vi "Main.vi"(11 "Module Admin":refnum<class "Delacor_lib_QMH_Module Admin.lvclass">) -> ()   [LabVIEW 2024, in "Settings Editor.lvlib"]
doc: "This template is based off of the Queued Message Handler design pattern and the Queued Message Handler project template that ships with LabVIEW.\n\nThe main difference is that the queue is private to this module and communication between modules is performed via Broadcast and Request events.\n\nRequest events are wrapped in public API methods and are handled in the Event Handling Loop (EHL) of this VI. Any module can register for Broadcast events sent by this module. The EHL generates messages based on user interface actions.\n\nThe Message Handling Loop (MHL) processes messages generated by the EHL, or by other messages. The messages are string values, so new messages can be added easily to the Message Cases case structure in the MHL. Each message cluster can also provide an optional value for Message Data, which is a variant that can be converted to whatever message-specific data is required.\n_____\nBased on DQMH Project Template 4.0.0.47.\n_____\nBased on DQMH Dev Tools: Project Template 7.1.0.1503."
uses:
  Settings Editor.lvlib
  <vilib>/Delacor/Delacor QMH/Libraries/Module Admin_class/Delacor_lib_QMH_Module Admin.lvclass
  CML Shared/Signal Type--enum.ctl
  CML Shared/Calibration Values--cluster.ctl
  Module Data--cluster.ctl
  Settings--cluster.ctl
  Stop Argument--cluster.ctl
  <vilib>/Delacor/Delacor QMH/Libraries/Message Queue_class/Delacor_lib_QMH_Message Queue.lvclass/Delacor_lib_QMH_Message Queue.ctl
  Update Application Settings Argument--cluster.ctl
  Update Application Settings (Reply Payload)--cluster.ctl
  <vilib>/Delacor/Delacor QMH/Libraries/Module Admin_class/Delacor_lib_QMH_Module Admin.lvclass/Delacor_lib_QMH_Module Admin.ctl
  <vilib>/Utility/miscctls.llb/LVPointTypeDef.ctl
  <vilib>/Delacor/Delacor QMH/Libraries/Message Queue_class/Delacor_lib_QMH_Enqueue Message (Single).vi
  <vilib>/Delacor/Delacor QMH/Libraries/Module Admin_class/Delacor_lib_QMH_Get External Launch.vi
  <vilib>/Delacor/Delacor QMH/Libraries/Message Queue_class/Delacor_lib_QMH_Message Queue.lvclass
  CML Shared/CML Shared.lvlib
panel:
  in  "Calibration Values":T1[](array[typedef])
  in  "Cancel":bool
  in  "OK":bool
  in  "Log File Base Path":path
  in  "Signal Type":T2
  out "error out":errorcluster
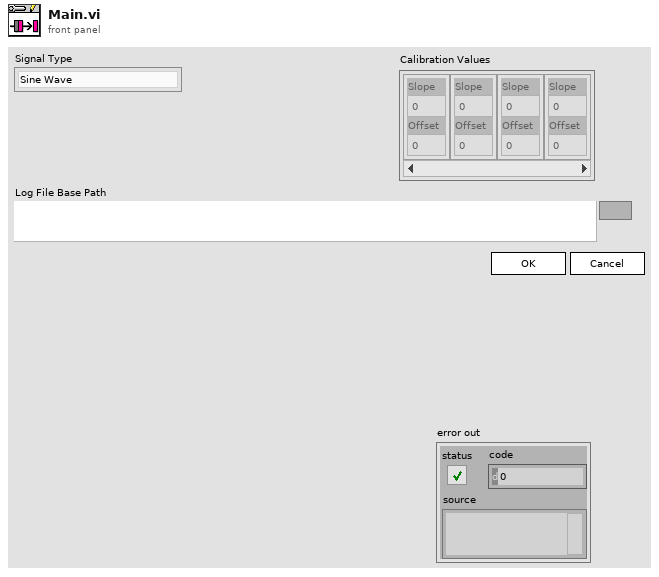
[diagram p1: front panel]
types:
  T1 = typedef "CML Shared.lvlib/Calibration Values--cluster.ctl" = cluster{"Slope":dbl, "Offset":dbl}
  T2 = typedef "CML Shared.lvlib/Signal Type--enum.ctl" = enum16{"Sine Wave", "Square with Noise"}
  T3 = typedef "Settings Editor.lvlib/Request Events--cluster.ctl" = cluster{"Stop Module":refnum<user-event>, "Show Panel":refnum<user-event>, "Hide Panel":refnum<user-event>, "Get Module Execution Status":refnum<user-event>, "Show Diagram":refnum<user-event>, "Update Application Settings":refnum<user-event>}
  T4 = typedef "Settings Editor.lvlib/Module Data--cluster.ctl" = cluster{"Settings":T5}
  T5 = typedef "Settings Editor.lvlib/Settings--cluster.ctl" = cluster{"Signal Type":T2, "Calibration Array":T1[], "Log File Base Path":path}
  T6 = enum32{"invalid lock state", "Not Locked", "Locked (No Password)", "Password-protected"}
  T7 = typedef "Settings Editor.lvlib/Stop Argument--cluster.ctl" = cluster{"Origin":string, "Exit via Stop Module Req?":bool, "Wait for Module to stop?":bool}
  T8 = typedef "Settings Editor.lvlib/Update Application Settings Argument--cluster.ctl" = cluster{"Wait Notifier":refnum<notifier>, "wait for reply":bool}
  T9 = typedef "LVPointTypeDef.ctl" = cluster{"Horizontal":i16, "Vertical":i16}
  T10 = enum32{"Invalid", "Standard", "Closed", "Hidden", "Minimized", "Maximized"}
  T11 = typedef "Settings Editor.lvlib/Update Application Settings (Reply Payload)--cluster.ctl" = cluster{"Settings":T5, "error":errorcluster}
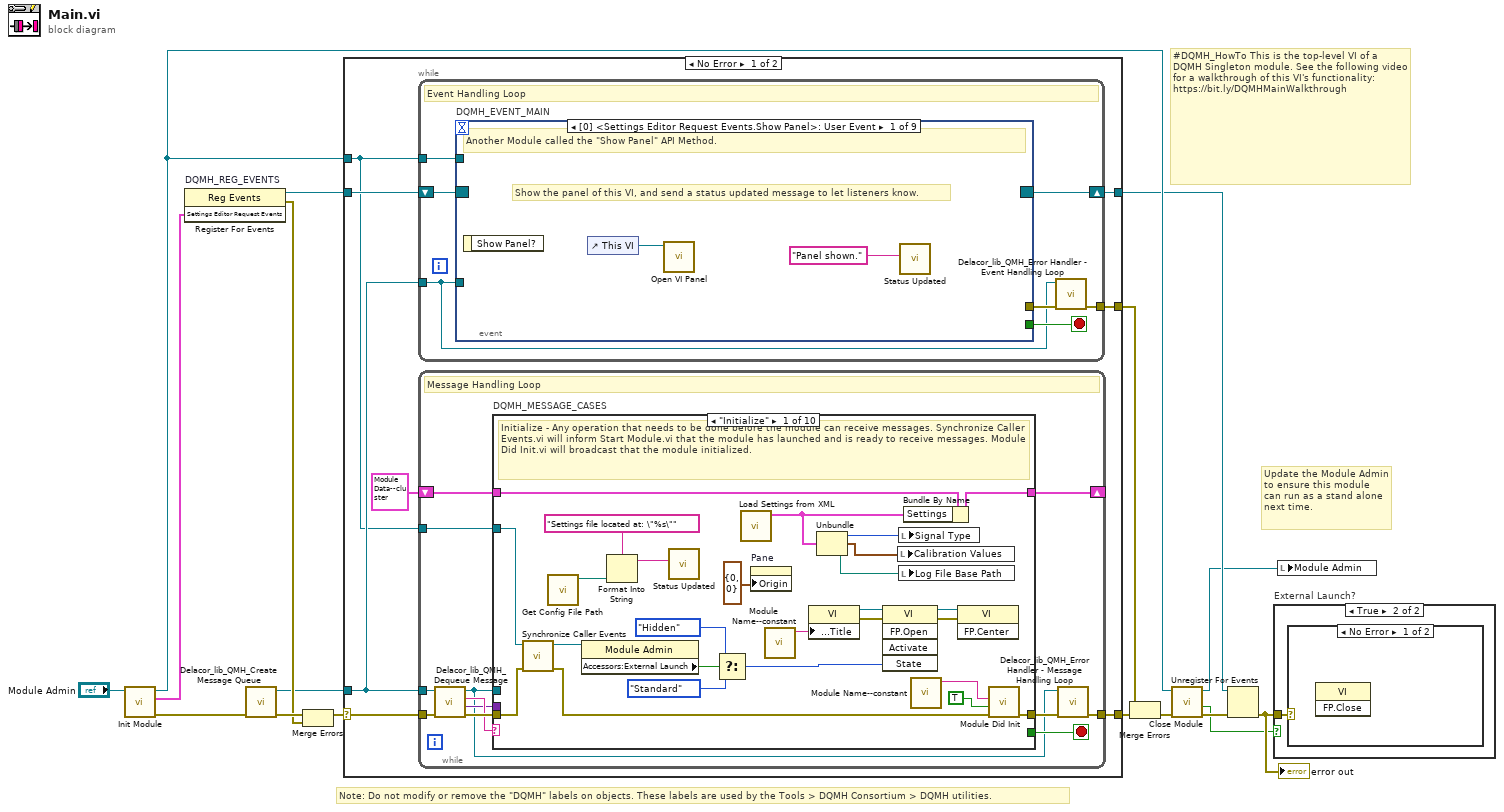
[diagram p0: block diagram]
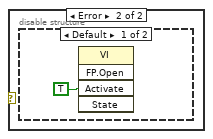
[diagram p3: hidden frame]
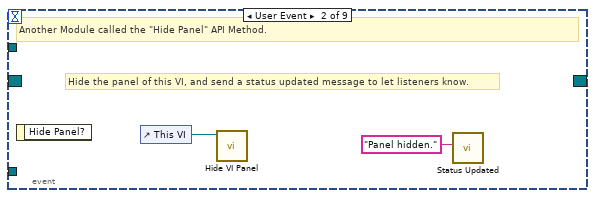
[diagram p5: hidden frame]
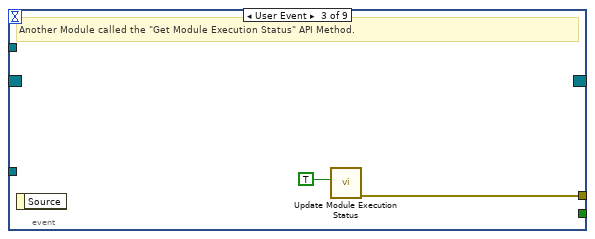
[diagram p6: hidden frame]
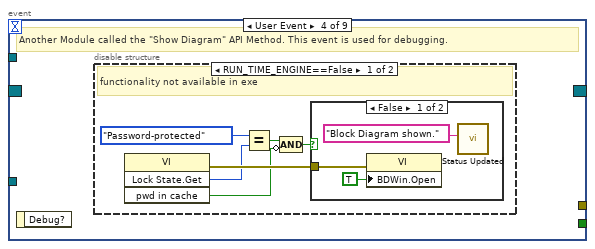
[diagram p7: hidden frame]
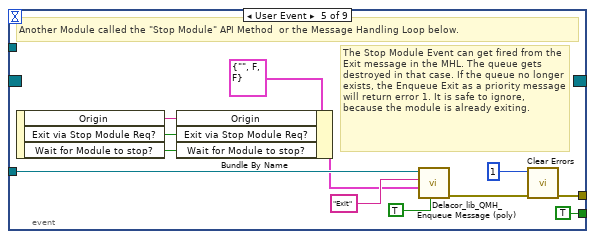
[diagram p10: hidden frame]
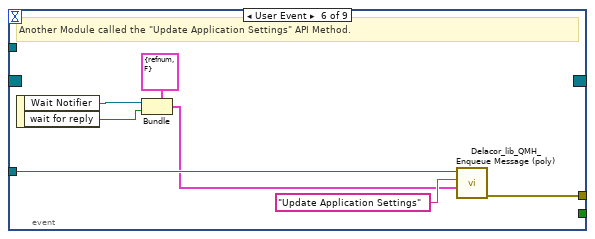
[diagram p11: hidden frame]
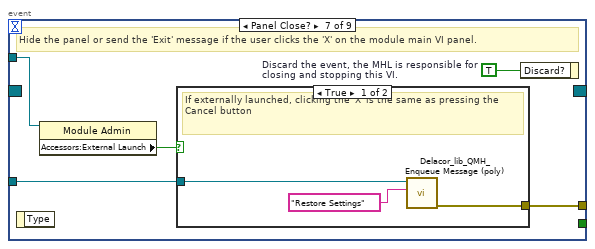
[diagram p12: hidden frame]
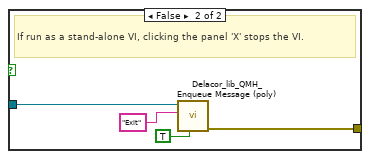
[diagram p13: hidden frame]
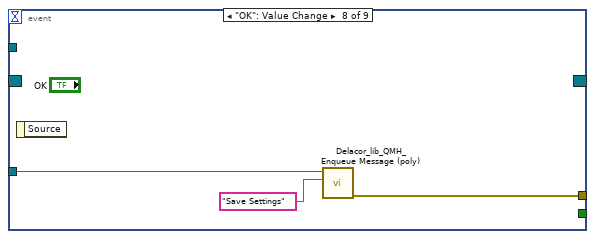
[diagram p14: hidden frame]
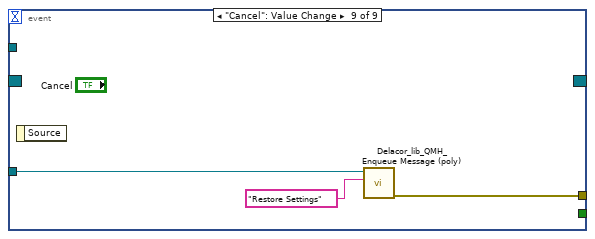
[diagram p15: hidden frame]
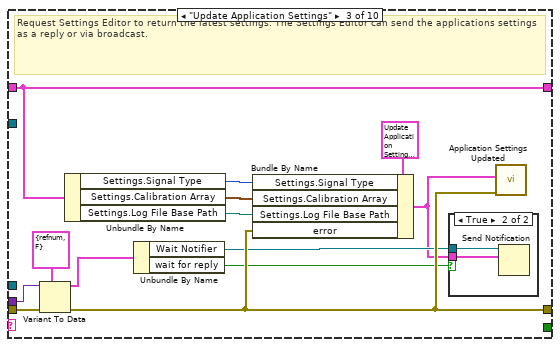
[diagram p17: hidden frame]
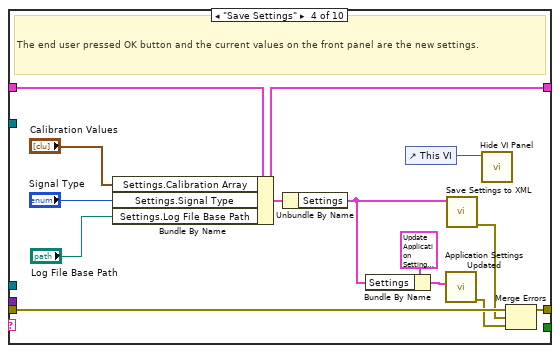
[diagram p19: hidden frame]
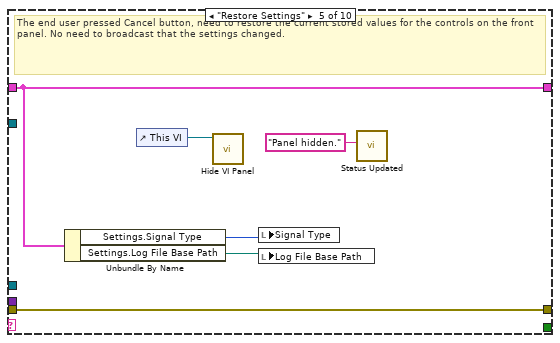
[diagram p20: hidden frame]
diagram:
  # "#DQMH_HowTo This is the top-level VI of a DQMH Singleton module. See the following video for a walkthrough of this VI's functionality: https://bit.ly/DQMHMainWalkthrough"
  # "Note: Do not modify or remove the \"DQMH\" labels on objects. These labels are used by the Tools > DQMH Consortium > DQMH utilities."
  # "Update the Module Admin to ensure this module can run as a stand alone next time."
  n1 = call "Init Module.vi"("Singleton Module Admin in"="Module Admin") -> ("error out"=w16:errorcluster, "Settings Editor Request Events"=w5:T3, "Singleton Module Admin out"=w8:refnum<class "Delacor_lib_QMH_Module Admin.lvclass">)  [unwired: 8 in]
  n2 = register-events "DQMH_REG_EVENTS"(w5) -> (reference out=w6:refnum<event-registration>, error out=w9:errorcluster)  [unwired: 2 in]
  n3 = call <vilib>:"Delacor_lib_QMH_Create Message Queue.vi"("error in"=w16) -> ("error out"=w11:errorcluster, "Message Queue"=w4:refnum<class "Delacor_lib_QMH_Message Queue.lvclass">)  [unwired: 9 in]
  n4 = Merge Errors(w11, w9) -> (w10:errorcluster)
  n5 = case shown="No Error" w10 {
    selector: w10 -> [w23 w213]
    tunnel: [w25 w212] -> w17
    tunnel: [w22 w211] -> w7
    tunnel: w6 -> [w20 w211]
    tunnel: w4 -> [w19 w206]
    tunnel: [w24 _] -> w14
    tunnel: w8 -> [w18 w207]
    frame No Error {
      n6 = while {
        tunnel: w19 -> [w26]
        shift-right: [w29] -> w22
        shift-left: w20 -> [w30]
        tunnel: [w31] -> w24
        tunnel: w18 -> [w27]
        stop <- w28 stop-if-true
        # "Event Handling Loop"
        n7 = event "DQMH_EVENT_MAIN" shown="[0] <Settings Editor Request Events.Show Panel>: User Event" {
          selector: w30 -> [_ _ _ _ _ _ _ _ _]
          dyn-events: [_ _ _ _ _ _ _ _ _] -> w29
          timeout: _ -> [_ _ _ _ _ _ _ _ _]
          tunnel: [_ _ _ _ TRUE ("Discard?") _ _ _ _] -> w28
          tunnel: w26 -> [_ _ _ _ w55 w65 w69 w79 w82]
          tunnel: [_ _ w38 _ w58 w66 w71 w81 w84] -> w32
          tunnel: w27 -> [_ _ _ _ _ _ w68 _ _]
          event User Event {
            # "Show the panel of this VI, and send a status updated message to let listeners know."
            # "Another Module called the \"Show Panel\" API Method."
            n8 = event-data() -> ()  [unwired: 1 in, 1 out]
            n9 = control-ref of="This VI"() -> (w34:refnum<vi>)
            n10 = call "Open VI Panel.vi"("VI"=w34) -> ()  [unwired: 10 in, 1 out]
            n11 = call "Status Updated.vi"("Status"="Panel shown." ("format string")) -> ()  [unwired: 10 in, 1 out]
          }
          event User Event {
            # "Hide the panel of this VI, and send a status updated message to let listeners know."
            # "Another Module called the \"Hide Panel\" API Method."
            n12 = event-data() -> ()  [unwired: 1 in, 1 out]
            n13 = control-ref of="This VI"() -> (w36:refnum<vi>)
            n14 = call "Hide VI Panel.vi"("VI"=w36) -> ()  [unwired: 10 in, 1 out]
            n15 = call "Status Updated.vi"("Status"="Panel hidden." ("format string")) -> ()  [unwired: 10 in, 1 out]
          }
          event User Event {
            # "Another Module called the \"Get Module Execution Status\" API Method."
            n16 = event-data() -> ()  [unwired: 1 in, 1 out]
            n17 = call "Update Module Execution Status.vi"("Running?"=TRUE) -> ("error out"=w38:errorcluster)  [unwired: 10 in]
          }
          event User Event {
            # "Another Module called the \"Show Diagram\" API Method. This event is used for debugging."
            n18 = event-data() -> ()  [unwired: 1 in, 1 out]
            n19 = disable-structure shown="RUN_TIME_ENGINE==False" {
              frame condition #0 (active) {
                # "functionality not available in exe"
                n20 = invoke on="Invoke Node" class="VI" method="Lock State.Get"() -> (error out=w44:errorcluster, "Get Lock State"=w43:T6, "pwd in cache"=w40:bool)  [unwired: 4 in, 1 out]
                n21 = Equal?(x=T6."Password-protected", y=w43) -> (x = y?=w41:bool)
                n22 = Compound Arithmetic op=AND(w41, invert w40) -> (w39:bool)
                n23 = case shown="False" w39 {
                  tunnel: w44 -> [w47 _]
                  frame False {
                    n24 = property on="Property Node" class="VI"(error in=w47, "BDWin.Open"=TRUE ("Block Diagram Window:Open")) -> ()  [unwired: 1 in, 2 out]
                    n25 = call "Status Updated.vi"("Status"="Block Diagram shown." ("format string")) -> ()  [unwired: 10 in, 1 out]
                  }
                  frame True {
                    # "Password-protected VI, and the password is not in the cache. Do not show the diagram."
                  }
                }
              }
              frame condition #1 {
              }
            }
          }
          event User Event {
            # "The Stop Module Event can get fired from the Exit message in the MHL. The queue gets destroyed in that case. If the queue no longer exists, the Enqueue Exit as a priority message will return error 1. It is safe to ignore, because the module is already exiting."
            # "Another Module called the \"Stop Module\" API Method  or the Message Handling Loop below."
            n26 = event-data() -> ("Origin"=w48:string, "Exit via Stop Module Req?"=w51:bool, "Wait for Module to stop?"=w50:bool)  [unwired: 1 in]
            n27 = Bundle By Name(cluster=T7 {"Origin"="", "Exit via Stop Module Req?"=FALSE, "Wait for Module to stop?"=FALSE} ("Stop Argument"), "Origin"=w48, "Exit via Stop Module Req?"=w51, "Wait for Module to stop?"=w50) -> (w49:T7)
            n28 = call-poly <vilib>:"Delacor_lib_QMH_Enqueue Message (poly).vi"("Priority Message? (F)"=TRUE, "Message Data"=w49, "Message"="Exit", "Message Queue in"=w55) -> ("error out"=w59:errorcluster)  [unwired: 6 in, 1 out]
            n29 = call <vilib>:"Clear Errors.vi"("error in (no error)"=w59, "specific error code to clear (0: all)"=1) -> ("error out"=w58:errorcluster)  [unwired: 4 in, 1 out]
          }
          event User Event {
            # "Another Module called the \"Update Application Settings\" API Method."
            n30 = event-data() -> ("Wait Notifier"=w61:refnum<notifier>, "wait for reply"=w60:bool)  [unwired: 1 in]
            n31 = Bundle(cluster=T8 {"Wait Notifier"=refnum, "wait for reply"=FALSE} ("Update Application Settings Argument"), "Wait Notifier"=w61, "wait for reply"=w60) -> (w62:T8)
            n32 = call-poly <vilib>:"Delacor_lib_QMH_Enqueue Message (poly).vi"("Message Data"=w62, "Message"="Update Application Settings", "Message Queue in"=w65) -> ("error out"=w66:errorcluster)  [unwired: 7 in, 1 out]
          }
          event Panel Close? {
            w70 = TRUE  # Discard the event, the MHL is responsible for closing and stopping this VI.
            # "Hide the panel or send the 'Exit' message if the user clicks the 'X' on the module main VI panel."
            n33 = event-data() -> ()  [unwired: 1 in, 1 out]
            n34 = property on="Property Node" class="Module Admin"(reference=w68) -> ("Accessors:External Launch"=w67:bool)  [unwired: 1 in, 2 out]
            n35 = case shown="True" w67 {
              tunnel: w69 -> [w72 w77]
              tunnel: [w74 w78] -> w71
              frame True {
                # "If externally launched, clicking the 'X' is the same as pressing the Cancel button"
                n36 = call-poly <vilib>:"Delacor_lib_QMH_Enqueue Message (poly).vi"("Message"="Restore Settings", "Message Queue in"=w72) -> ("error out"=w74:errorcluster)  [unwired: 8 in, 1 out]
              }
              frame False {
                # "If run as a stand-alone VI, clicking the panel 'X' stops the VI."
                n37 = call-poly <vilib>:"Delacor_lib_QMH_Enqueue Message (poly).vi"("Priority Message? (F)"=TRUE, "Message"="Exit", "Message Queue in"=w77) -> ("error out"=w78:errorcluster)  [unwired: 7 in, 1 out]
              }
            }
            n38 = event-data ("Event Filter Node")("Discard?"=w70) -> ()  [unwired: 1 in, 1 out]
          }
          event "OK": Value Change {
            n39 = event-data() -> ()  [unwired: 1 in, 1 out]
            n40 = call-poly <vilib>:"Delacor_lib_QMH_Enqueue Message (poly).vi"("Message"="Save Settings", "Message Queue in"=w79) -> ("error out"=w81:errorcluster)  [unwired: 8 in, 1 out]
          }
          event "Cancel": Value Change {
            n41 = event-data() -> ()  [unwired: 1 in, 1 out]
            n42 = call-poly <vilib>:"Delacor_lib_QMH_Enqueue Message (poly).vi"("Message"="Restore Settings", "Message Queue in"=w82) -> ("error out"=w84:errorcluster)  [unwired: 8 in, 1 out]
          }
        }
        n43 = call-dynamic "Delacor_lib_QMH_Error Handler - Event Handling Loop.vi"("error in"=w32, "Message Queue in"=w26) -> ("dup error in"=w31:errorcluster)  [unwired: 8 in, 1 out]
      }
      n44 = while {
        tunnel: w19 -> [w87]
        shift-right: [w91] -> _
        shift-left: T4 {"Settings"={"Signal Type"=enum."Sine Wave", "Calibration Array"=[{"Slope"=1.0, "Offset"=0.0}], "Log File Base Path"=path ""}} ("Data Cluster") -> [w92]
        tunnel: w23 -> [w95]
        tunnel: [w93] -> w25
        tunnel: w18 -> [w85]
        stop <- w90 stop-if-true
        # "Message Handling Loop"
        n45 = call-dynamic "Delacor_lib_QMH_Dequeue Message.vi"("error in"=w95, "Message Queue in"=w87) -> ("error out"=w94:errorcluster, "Message Data"=w88:variant, "Message"=w89:string, "Message Queue out"=w86:refnum<class "Delacor_lib_QMH_Message Queue.lvclass">)  [unwired: 6 in]
        n46 = case "DQMH_MESSAGE_CASES" shown="\"Initialize\"" w89 {
          selector: w89 -> [_ _ _ _ _ _ _ _ _ w201]
          tunnel: w86 -> [_ _ _ _ _ _ _ w167 w189 _]
          tunnel: w94 -> [w121 w124 w136 w151 w158 w161 w163 w174 w195 w204]
          tunnel: [w119 w124 w137 w152 w158 w160 w163 w170 w190 w205] -> w96
          tunnel: w92 -> [w109 w123 w130 w148 w157 w159 w162 w169 w188 w202]
          tunnel: [w108 w123 w130 w145 w157 w159 w162 w169 w188 w202] -> w91
          tunnel: [_ _ _ _ _ _ _ _ w187 _] -> w90
          tunnel: w88 -> [_ _ w135 _ _ _ _ w168 w186 _]
          tunnel: w85 -> [w110 _ _ _ _ _ _ w166 w181 _]
          frame "Initialize" {
            # "Initialize - Any operation that needs to be done before the module can receive messages. Synchronize Caller Events.vi will inform Start Module.vi that the module has launched and is ready to receive messages. Module Did Init.vi will broadcast that the module initialized."
            n47 = call "Synchronize Caller Events.vi"("error in"=w121, "Singleton Module Admin in"=w110) -> ("error out"=w120:errorcluster, "Singleton Module Admin out"=w105:refnum<class "Delacor_lib_QMH_Module Admin.lvclass">)  [unwired: 8 in]
            n48 = call "Get Config File Path.vi"() -> ("XML File Path"=w103:path)  [unwired: 10 in, 1 out]
            n49 = property on="Property Node" class="Module Admin"(reference=w105) -> ("Accessors:External Launch"=w114:bool)  [unwired: 1 in, 2 out]
            n50 = Format Into String(format string="Settings file located at: \"%s\"", w103) -> (resulting string=w102:string)  [unwired: 2 in, 1 out]
            n51 = call "Status Updated.vi"("Status"=w102) -> ()  [unwired: 10 in, 1 out]
            n52 = Select(t=T10."Hidden" ("State"), s=w114, f=T10."Standard" ("State")) -> (s? t:f=w111:T10)
            n53 = call "Load Settings from XML.vi"() -> ("Settings out"=w100:T5)  [unwired: 10 in, 1 out]
            n54 = property on="Pane" class="Pane"("Origin"=T9 {"Horizontal"=0, "Vertical"=0}) -> ()  [unwired: 2 in, 2 out]
            n55 = call "Module Name--constant.vi"() -> ("Module Name"=w117:string)  [unwired: 11 in]
            n56 = property on="Property Node" class="VI"("Front Panel.Title"=w117) -> (reference out=w116:refnum<vi>, error out=w118:errorcluster)  [unwired: 2 in]
            n57 = Unbundle(w100) -> ("Signal Type"=w99:T2, "Calibration Array"=w98:T1[], "Log File Base Path"=w97:path)
            n58 = invoke on="Invoke Node" class="VI" method="FP.Open"(reference=w116, error in=w118, "State"=w111) -> (reference out=w115:refnum<vi>, error out=w122:errorcluster)  [unwired: 2 in, 3 out]
            n59 = local write "Calibration Values"(w98) -> ()
            n60 = local write "Signal Type"(w99) -> ()
            n61 = local write "Log File Base Path"(w97) -> ()
            n62 = Bundle By Name(cluster=w109, "Settings"=w100) -> (w108:T4)
            n63 = call "Module Name--constant.vi"() -> ("Module Name"=w106:string)  [unwired: 11 in]
            n64 = invoke on="Invoke Node" class="VI" method="FP.Center"(reference=w115, error in=w122) -> ()  [unwired: 1 in, 3 out]
            n65 = call "Module Did Init.vi"("error in"=w120, "Initialized?"=TRUE, "Origin"=w106) -> ("error out"=w119:errorcluster)  [unwired: 8 in]
          }
          frame "---Module Specific---" {
            # "Separator -- The following cases handle messages specific to this Module."
          }
          frame "Update Application Settings" {
            # "Request Settings Editor to return the latest settings. The Settings Editor can send the applications settings as a reply or via broadcast."
            n66 = Variant To Data(error in=w136, type=T8 {"Wait Notifier"=refnum, "wait for reply"=FALSE} ("Update Application Settings Argument"), Variant=w135) -> (data=w133:T8, error out=w137:errorcluster)
            n67 = Unbundle By Name(w130) -> ("Settings.Signal Type"=w128:T2, "Settings.Calibration Array"=w127:T1[], "Settings.Log File Base Path"=w126:path)
            n68 = Unbundle By Name(w133) -> ("Wait Notifier"=w132:refnum<notifier>, "wait for reply"=w131:bool)
            n69 = Bundle By Name(cluster=T11 {"Settings"={"Signal Type"=enum."Sine Wave", "Calibration Array"=[], "Log File Base Path"=path ""}, "error"={"status"=FALSE, "code"=0, "source"=""}} ("Update Application Settings (Reply Payload)"), "Settings.Signal Type"=w128, "Settings.Calibration Array"=w127, "Settings.Log File Base Path"=w126, "error"=w137) -> (w125:T11)
            n70 = case shown="True" w131 {
              tunnel: w132 -> [_ w139]
              tunnel: w125 -> [_ w138]
              frame False {
              }
              frame True {
                n71 = Send Notification(notification=w138, notifier=w139) -> ()  [unwired: 1 in, 2 out]
              }
            }
            n72 = call "Application Settings Updated.vi"("error in"=w137, "Reply Payload"=w125) -> ()  [unwired: 9 in, 1 out]
          }
          frame "Save Settings" {
            # "The end user pressed OK button and the current values on the front panel are the new settings."
            n73 = Bundle By Name(cluster=w148, "Settings.Calibration Array"="Calibration Values", "Settings.Signal Type"="Signal Type", "Settings.Log File Base Path"="Log File Base Path") -> (w145:T4)
            n74 = Unbundle By Name(w145) -> ("Settings"=w140:T5)
            n75 = Bundle By Name(cluster=T11 {"Settings"={"Signal Type"=enum."Sine Wave", "Calibration Array"=[], "Log File Base Path"=path ""}, "error"={"status"=FALSE, "code"=0, "source"=""}} ("Reply Payload"), "Settings"=w140) -> (w141:T11)
            n76 = control-ref of="This VI"() -> (w146:refnum<vi>)
            n77 = call "Application Settings Updated.vi"("Reply Payload"=w141) -> ("error out"=w149:errorcluster)  [unwired: 10 in]
            n78 = call "Save Settings to XML.vi"("Settings"=w140) -> ("error out"=w150:errorcluster)  [unwired: 10 in]
            n79 = call "Hide VI Panel.vi"("VI"=w146) -> ()  [unwired: 10 in, 1 out]
            n80 = Merge Errors(w151, w150, w149) -> (w152:errorcluster)
          }
          frame "Restore Settings" {
            # "The end user pressed Cancel button, need to restore the current stored values for the controls on the front panel. No need to broadcast that the settings changed."
            n81 = Unbundle By Name(w157) -> ("Settings.Signal Type"=w156:T2, "Settings.Log File Base Path"=w155:path)
            n82 = control-ref of="This VI"() -> (w154:refnum<vi>)
            n83 = call "Hide VI Panel.vi"("VI"=w154) -> ()  [unwired: 10 in, 1 out]
            n84 = local write "Signal Type"(w156) -> ()
            n85 = local write "Log File Base Path"(w155) -> ()
            n86 = call "Status Updated.vi"("Status"="Panel hidden." ("format string")) -> ()  [unwired: 10 in, 1 out]
          }
          frame "---Copy This Frame---" {
            # "Duplicate this frame when creating new messages.  Change this comment in the duplicated frame to describe this message."
            n87 = Merge Errors(w161) -> (w160:errorcluster)
          }
          frame "---Exit and Error Handling---" {
            # "Separator - The following cases handle errors and exit messages."
          }
          frame "Error" {
            # "Error - Check the error message data and respond accordingly. This message is sent by the \"Error Handler\" VIs at the end of each loop in this application."
            n88 = property on="Property Node" class="Module Admin"(reference=w166) -> ("Accessors:External Launch"=w165:bool)  [unwired: 1 in, 2 out]
            n89 = Variant To Data(error in=w174, type=errorcluster {"status"=FALSE, "code"=0, "source"=""} ("error constant"), Variant=w168) -> (data=w164:errorcluster, error out=w172:errorcluster)
            n90 = local write "error out"(w164) -> ()
            n91 = call "Error Reported.vi"("Error"=w164) -> ()  [unwired: 10 in, 1 out]
            n92 = case shown="False" w165 {
              tunnel: [w179 _] -> w171
              tunnel: w167 -> [w177 _]
              tunnel: w164 -> [w178 _]
              frame False {
                n93 = disable-structure shown="Default" {
                  disable-tunnel: w178 -> [w180 _]
                  frame condition #0 (active) {
                    # "If the module is running standalone, then pop up an error dialog and call the \"Exit\" message."
                    n94 = call <vilib>:"Simple Error Handler.vi"("error in (no error)"=w180) -> ()  [unwired: 4 in, 5 out]
                  }
                  frame condition #1 {
                    # "To prevent the Simple Error Handler VI from being loaded (e.g. when deploying to a Real-Time target), add the Conditional Disable Symbol \"DQMH_Disable_SEH\" to your project and set it to TRUE."
                  }
                }
                n95 = call-poly <vilib>:"Delacor_lib_QMH_Enqueue Message (poly).vi"("Priority Message? (F)"=TRUE, "Message"="Exit", "Message Queue in"=w177) -> ("error out"=w179:errorcluster)  [unwired: 7 in, 1 out]
              }
              frame True {
                # "If the module was launched externally, calling the Error Reported broadcast VI is the only action performed by the \"Error\" message. The module's caller can then process the error appropriately."
              }
            }
            n96 = Merge Errors(w172, w171) -> (w170:errorcluster)
          }
          frame "Exit" {
            w187 = TRUE  # Stop the VI
            # "Release the message queue reference"
            # "Exit - Exit the application."
            n97 = Variant To Data(error in=w195, type=T7 {"Origin"="", "Exit via Stop Module Req?"=FALSE, "Wait for Module to stop?"=FALSE} ("Stop Argument"), Variant=w186) -> (data=w183:T7, error out=w192:errorcluster)
            n98 = call <vilib>:"Clear Errors.vi"("error in (no error)"=w192, "specific error code to clear (0: all)"=91 ("91: not all Exit messages will have an argument")) -> ("error out"=w194:errorcluster)  [unwired: 4 in, 1 out]
            n99 = control-ref of="This VI"() -> (w182:refnum<vi>)
            n100 = call-dynamic "Delacor_lib_QMH_Release Message Queue.vi"("error in"=w194, "Message Queue"=w189) -> ("error out"=w193:errorcluster)  [unwired: 9 in]
            n101 = call "Handle Exit.vi"("Stop Argument"=w183, "Admin in"=w181, "VI reference"=w182) -> ("error out"=w191:errorcluster)  [unwired: 7 in, 1 out]
            n102 = Merge Errors(w193, w191) -> (w190:errorcluster)
            n103 = call "Error Reported.vi"("Error"=w190) -> ()  [unwired: 10 in, 1 out]
          }
          frame Default {
            # "'Default' case only runs if there is a message that isn't defined in any of the other cases.  Output a programming error."
            n104 = call "Module Name--constant.vi"() -> ("Module Name"=w200:string)  [unwired: 11 in]
            n105 = Format Into String(format string="The invalid message string \"%s\" was received in the Message Handling Loop for module \"%s\".", w201, w200) -> (resulting string=w198:string)  [unwired: 2 in, 1 out]
            n106 = call <vilib>:"Error Cluster From Error Code.vi"("show call chain? (False)"=TRUE, "error message (\"\")"=w198, "error code (0)"=1) -> ("error out"=w203:errorcluster)  [unwired: 6 in]
            n107 = Merge Errors(w204, w203) -> (w205:errorcluster)
          }
        }
        n108 = call-dynamic "Delacor_lib_QMH_Error Handler - Message Handling Loop.vi"("error in"=w96, "Message Queue in"=w86) -> ("dup error in"=w93:errorcluster)  [unwired: 8 in, 1 out]
      }
    }
    frame Error {
      # "Synchronize Caller Events.vi will inform Start Module.vi that the module has launched and will let the code calling Start Module.vi register for broadcasts and would permit the caller receive the broadcast that an error occurred at launch time."
      n109 = call "Synchronize Caller Events.vi"("Singleton Module Admin in"=w207) -> ("error out"=w214:errorcluster)  [unwired: 9 in, 1 out]
      n110 = call-dynamic "Delacor_lib_QMH_Release Message Queue.vi"("error in"=w213, "Message Queue"=w206) -> ("error out"=w212:errorcluster)  [unwired: 9 in]
      n111 = call "Module Name--constant.vi"() -> ("Module Name"=w210:string)  [unwired: 11 in]
      n112 = Format Into String(format string="An error occurred during initialization. %s is no longer running.", w210) -> (resulting string=w208:string)  [unwired: 2 in, 1 out]
      n113 = Merge Errors(w212, w214) -> (w215:errorcluster)
      n114 = call "Error Reported.vi"("Additional Information"=w208, "Error"=w215) -> ()  [unwired: 9 in, 1 out]
    }
  }
  n115 = Merge Errors(w14, w17) -> (w13:errorcluster)
  n116 = call "Close Module.vi"("error in"=w13, "Module Admin in"=w8) -> ("error out"=w15:errorcluster, "External Launch"=w1:bool, "Module Admin out"=w2:refnum<class "Delacor_lib_QMH_Module Admin.lvclass">)  [unwired: 7 in]
  n117 = Unregister For Events(event registration refnum=w7, error in=w15) -> (error out=w12:errorcluster)
  "error out" <- w12
  n118 = case "External Launch?" shown="True" w1 {
    tunnel: w12 -> [_ w216]
    frame False {
    }
    frame True {
      n119 = case shown="No Error" w216 {
        frame No Error {
          n120 = invoke on="Invoke Node" class="VI" method="FP.Close"() -> ()  [unwired: 3 in, 3 out]
        }
        frame Error {
          n121 = disable-structure shown="Default" {
            frame condition #0 (active) {
              n122 = invoke class="VI" method="FP.Open"("Activate"=TRUE ("Activate?")) -> ()  [unwired: 4 in, 5 out]
            }
            frame condition #1 {
              # "Don't show panel on error if running inside a built EXE."
            }
          }
        }
      }
    }
  }
  n123 = local write "Module Admin"(w2) -> ()
